vi "Err vs Lock Size Real.vi"() -> ()   [LabVIEW 2016]
panel:
  in  "frac":dbl
  out "XY Graph":cluster{"X":dbl, "Y":dbl}[](graph)=[{"X"=-0.1, "Y"=26.830233276198005}, {"X"=-0.1, "Y"=26.76099227793343}, {"X"=-0.0999, "Y"=26.962041822703505}, {"X"=-0.0997, "Y"=26.859853175835706}, {"X"=-0.0994, "Y"=26.741575418923244}, {"X"=-0.099, "Y"=26.75684267676379}, {"X"=-0.0985, "Y"=26.835573156776707}, {"X"=-0.0979, "Y"=26.714281352249014}, {"X"=-0.0972, "Y"=26.882117386451412}, {"X"=-0.0964, "Y"=26.791838062147157}, {"X"=-0.0955, "Y"=26.776249077595264}, {"X"=-0.0945, "Y"=26.90056616966124}, {"X"=-0.0934, "Y"=26.7876512849999}, {"X"=-0.09219999999999999, "Y"=26.782645192201798}, {"X"=-0.0909, "Y"=26.61806532920592}, {"X"=-0.0895, "Y"=26.737804547389686}, {"X"=-0.088, "Y"=26.634554337702188}, {"X"=-0.08639999999999999, "Y"=26.62053912929272}, {"X"=-0.0847, "Y"=26.553688543829054}, {"X"=-0.0829, "Y"=26.56494713578414}, {"X"=-0.081, "Y"=26.616344873323055}, {"X"=-0.079, "Y"=26.51641064776968}, {"X"=-0.0769, "Y"=26.447290055082522}, {"X"=-0.0747, "Y"=26.537349996332228}, {"X"=-0.0724, "Y"=26.379368428195058}, {"X"=-0.07, "Y"=26.321833093975314}, {"X"=-0.0675, "Y"=26.37673545704292}, {"X"=-0.0649, "Y"=26.32326061469585}, {"X"=-0.0622, "Y"=26.38181105483659}, {"X"=-0.0594, "Y"=26.18261725610268}, {"X"=-0.0565, "Y"=26.263610223129618}, {"X"=-0.0535, "Y"=26.148394502729534}, {"X"=-0.0504, "Y"=26.22179968801735}, {"X"=-0.0472, "Y"=26.161847256731598}, {"X"=-0.0439, "Y"=26.03355018880131}, {"X"=-0.0405, "Y"=26.095954862143014}, {"X"=-0.037, "Y"=26.02926093091044}, {"X"=-0.0334, "Y"=25.915662729989023}, {"X"=-0.029699999999999997, "Y"=26.01674232418862}, {"X"=-0.025899999999999996, "Y"=25.973269518710826}, {"X"=-0.021999999999999995, "Y"=25.962124237931082}, {"X"=-0.017999999999999995, "Y"=25.904856573895664}, {"X"=-0.013899999999999996, "Y"=25.78308669923812}, {"X"=-0.009699999999999995, "Y"=25.940673408056117}, {"X"=-0.005399999999999995, "Y"=25.976109421405802}, {"X"=-0.0009999999999999948, "Y"=26.00248549580469}, {"X"=0.0035000000000000057, "Y"=25.812625541764564}, {"X"=0.008100000000000007, "Y"=25.775406013461634}, {"X"=0.012800000000000006, "Y"=25.990697925850252}, {"X"=0.017600000000000005, "Y"=25.942630451311206}, {"X"=0.022500000000000006, "Y"=25.970767666952465}, {"X"=0.027500000000000007, "Y"=26.053081657887994}, {"X"=0.032600000000000004, "Y"=25.99996284838727}, {"X"=0.03780000000000001, "Y"=26.084903634177092}, {"X"=0.043100000000000006, "Y"=25.9704045671558}, {"X"=0.04850000000000001, "Y"=25.98704631231145}, {"X"=0.054000000000000006, "Y"=26.07454954761314}, {"X"=0.05960000000000001, "Y"=26.144657703616602}, {"X"=0.06530000000000001, "Y"=26.283721698995738}, {"X"=0.07110000000000001, "Y"=26.299036774020237}, {"X"=0.07700000000000001, "Y"=26.482307571762284}, {"X"=0.08300000000000002, "Y"=26.535199512754076}, {"X"=0.08910000000000001, "Y"=26.549310013354525}, {"X"=0.09530000000000001, "Y"=26.711028768013193}, {"X"=0.10160000000000001, "Y"=26.801387374821328}, {"X"=0.10800000000000001, "Y"=26.877498025784345}, {"X"=0.11450000000000002, "Y"=26.98785964565474}, {"X"=0.12110000000000001, "Y"=27.092058876623966}, {"X"=0.12780000000000002, "Y"=27.286022502298685}, {"X"=0.13460000000000003, "Y"=27.45193506545341}, {"X"=0.14150000000000001, "Y"=27.471128839286248}, {"X"=0.14850000000000002, "Y"=27.644305997597346}, {"X"=0.15560000000000002, "Y"=27.710308129481945}, {"X"=0.16280000000000003, "Y"=28.041305322411894}, {"X"=0.17010000000000003, "Y"=28.108502638666724}, {"X"=0.17750000000000002, "Y"=28.1982452579574}, {"X"=0.18500000000000003, "Y"=28.327270531167905}, {"X"=0.19260000000000002, "Y"=28.50200043204823}, {"X"=0.20030000000000003, "Y"=28.957073526014803}, {"X"=0.20810000000000003, "Y"=29.09876986021467}, {"X"=0.21600000000000003, "Y"=29.326743310321422}, {"X"=0.22400000000000003, "Y"=29.24035978004302}, {"X"=0.23210000000000003, "Y"=29.64528942912991}, {"X"=0.24030000000000004, "Y"=29.84336286601284}, {"X"=0.24860000000000004, "Y"=30.043786614895815}, {"X"=0.25700000000000006, "Y"=30.239049669962778}, {"X"=0.26550000000000007, "Y"=30.435185251838107}, {"X"=0.27410000000000007, "Y"=30.79803108832678}, {"X"=0.28280000000000005, "Y"=30.796890517111457}, {"X"=0.2916, "Y"=31.15754638183768}, {"X"=0.30050000000000004, "Y"=31.411359384361837}, {"X"=0.30950000000000005, "Y"=31.656637189151336}, {"X"=0.31860000000000005, "Y"=31.96343881817744}, {"X"=0.32780000000000004, "Y"=32.25280898036743}, {"X"=0.3371, "Y"=32.532378093917366}, {"X"=0.34650000000000003, "Y"=32.6701293003864}, {"X"=0.35600000000000004, "Y"=33.03294163697936}, {"X"=0.36560000000000004, "Y"=33.17347947707888}, {"X"=0.3753, "Y"=33.526658382506966}, {"X"=0.3851, "Y"=33.76228154807898}, {"X"=0.395, "Y"=34.19367689379211}, {"X"=0.405, "Y"=34.5051359468715}, {"X"=0.4151, "Y"=34.69469061177939}, {"X"=0.4253, "Y"=35.165036757711874}, {"X"=0.4356, "Y"=35.407172220035704}, {"X"=0.446, "Y"=35.6447384493488}, {"X"=0.4565, "Y"=35.91433224436365}, {"X"=0.4671, "Y"=36.21200630217285}, {"X"=0.4778, "Y"=36.63161060850592}, {"X"=0.4886, "Y"=36.90043774198649}, {"X"=0.4995, "Y"=37.21760250783779}]
  in  "dfrac":dbl=0.0001
  in  "frac max":dbl=0.5
  in  "frac min":dbl=-0.1
  in  "Array":cluster{"Vsg":dbl[], "B":dbl[]}[](array[cluster])=[{"Vsg"=[0.14, 0.31, 0.42, 0.55], "B"=[4.0, 6.0, 8.0, 9.0]}, {"Vsg"=[0.22, 0.31, 0.42, 0.48], "B"=[4.0, 6.0, 8.0, 9.0]}, {"Vsg"=[0.28, 0.31, 0.42, 0.43], "B"=[4.0, 6.0, 8.0, 9.0]}]
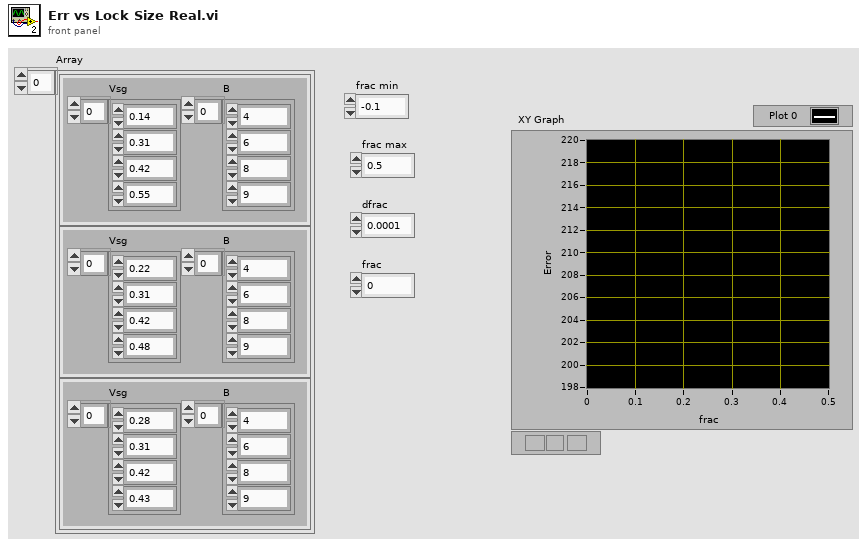
[diagram p1: front panel]
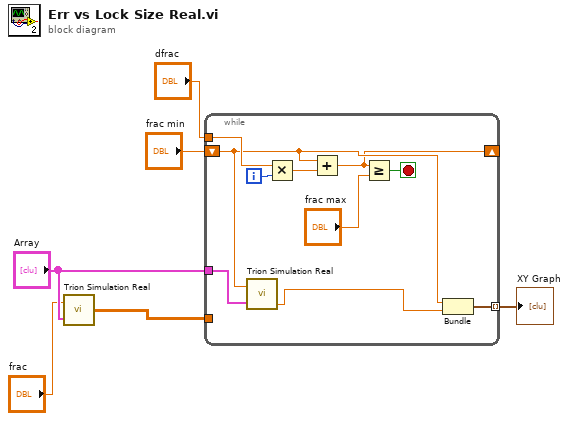
[diagram p0: block diagram]
diagram:
  n1 = call "Trion Simulation Real.vi"("frac"="frac", "Array"="Array") -> ("Fit"=w3:dbl[][])  [unwired: 2 out]
  n2 = while {
    shift-right: [w8] -> _
    shift-left: "frac min" -> [w10]
    tunnel: "dfrac" -> [w16]
    tunnel: "Array" -> [w11]
    tunnel: w3 -> [_]
    tunnel: [w9] -> w2 mode=indexing
    i -> [w15]
    stop <- w12 stop-if-true
    n3 = call "Trion Simulation Real.vi"("frac"=w10, "Array"=w11) -> ("err"=w7:dbl)  [unwired: 2 out]
    n4 = Multiply(x=w16, y=w15) -> (x*y=w14:dbl)
    n5 = Add(x=w10, y=w14) -> (x+y=w8:dbl)
    n6 = Greater Or Equal?(x=w8, y="frac max") -> (x >= y?=w12:bool)
    n7 = Bundle("frac min"=w10, "err"=w7) -> (w9:cluster{"frac min":dbl, "err":dbl})  [unwired: 1 in]
  }
  "XY Graph" <- w2
